vi "4-2-1 Chemical Process Monitoring.vi"() -> ()   [LabVIEW 2020]
uses:
  state.ctl
  <vilib>/addons/WebSockets-API-master/WebSockets/WebSocket Client/WebSocket Client.lvclass
  C:/Program Files (x86)/National Instruments/LabVIEW 2020/vi.lib/addons/WebSockets-API-master/WebSockets/WebSocket/WebSocket.lvclass
  <vilib>/addons/WebSockets-API-master/WebSockets/WebSocket/WebSocket.lvclass
panel:
  out "Read Data":string
  in  "Stop":bool
  out "connection error?":bool
  in  "sensor_data":T1={"temp_reactor"=60.0, "temp_coolant"=25.0, "press_reactor"=1.2, "stir_speed"=220.0, "coolant_flow"=TRUE, "exhaust_valve"=FALSE, "timestamp"="21:38:10"}
  out "connect?":bool
  in  "WebSockets URL":string="ws://localhost:8000/ws/labview"
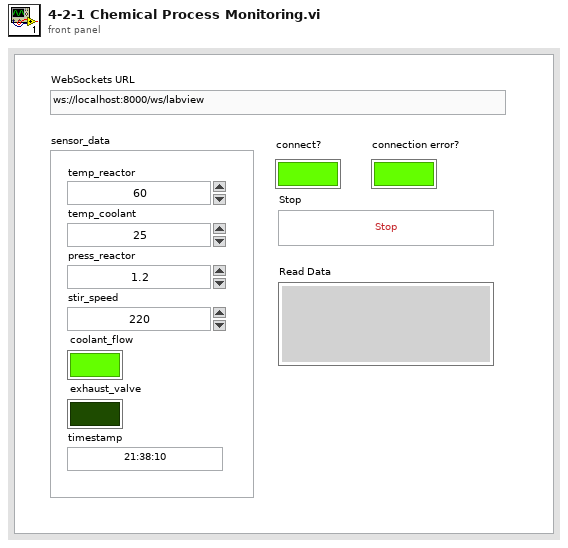
[diagram p1: front panel]
types:
  T1 = cluster{"temp_reactor":dbl, "temp_coolant":dbl, "press_reactor":dbl, "stir_speed":dbl, "coolant_flow":bool, "exhaust_valve":bool, "timestamp":string}
  T2 = typedef "state.ctl" = enum16{"CONNECT", "WRITE_DATA", "READ_DATA", "DISCONNECT"}
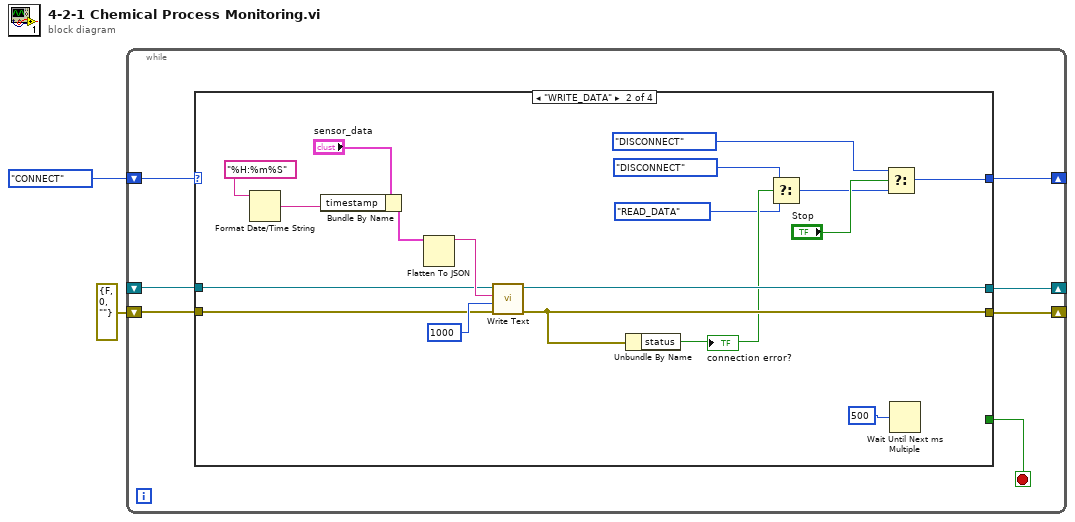
[diagram p0: block diagram]
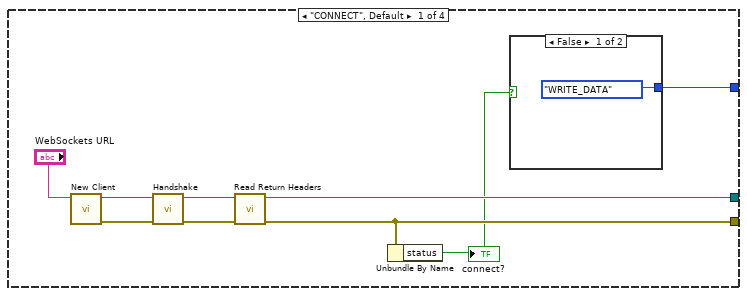
[diagram p2: hidden frame]
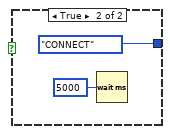
[diagram p3: hidden frame]
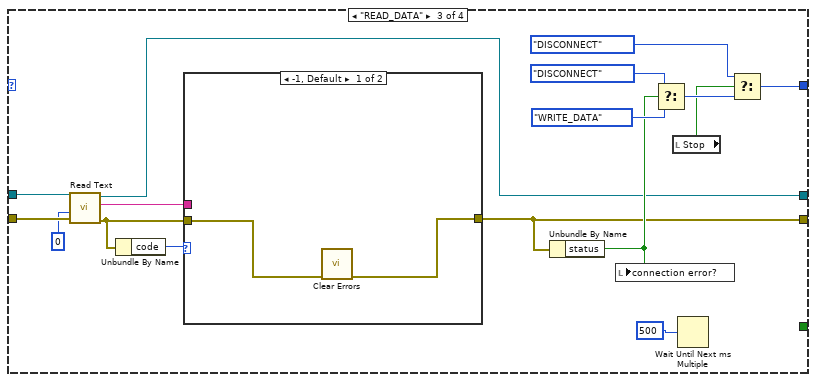
[diagram p4: hidden frame]
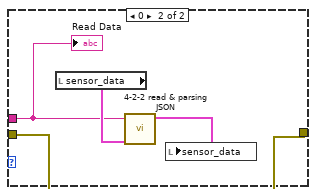
[diagram p5: hidden frame]
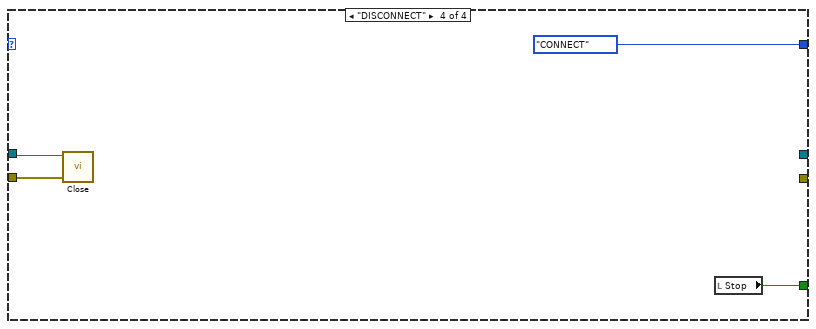
[diagram p6: hidden frame]
diagram:
  n1 = while {
    shift-right: [w6] -> _
    shift-left: state."CONNECT" -> [w9]
    shift-right: [w8] -> _
    shift-left: _ -> [w5]
    shift-right: [w7] -> _
    shift-left: errorcluster {"status"=FALSE, "code"=0, "source"=""} ("error out") -> [w4]
    stop <- w3 stop-if-true
    n2 = case shown="\"WRITE_DATA\"" w9 {
      tunnel: [w13 w35 w41 _] -> w8
      tunnel: [w12 w34 w42 _] -> w7
      tunnel: [w10 w26 w51 state."CONNECT"] -> w6
      tunnel: w5 -> [_ w37 w48 w65]
      tunnel: w4 -> [_ w36 w47 w64]
      tunnel: [_ _ _ w63] -> w3
      frame "CONNECT", Default {
        n3 = call <vilib>:"New Client.vi"("WebSocket URL"="WebSockets URL") -> ("error out"=w14:errorcluster, "WebSocket Client out"=w16:refnum<class "WebSocket Client.lvclass">)  [unwired: 9 in]
        n4 = call-dynamic "Handshake.vi"("error in (no error)"=w14, "WebSocket Client in"=w16) -> ("error out"=w17:errorcluster, "WebSocket Client out"=w18:refnum<class "WebSocket Client.lvclass">)  [unwired: 8 in]
        n5 = call <vilib>:"Read Return Headers.vi"("error in (no error)"=w17, "WebSocket in"=w18) -> ("error out"=w12:errorcluster, "WebSocket out"=w13:refnum<class "WebSocket Client.lvclass">)  [unwired: 7 in, 1 out]
        n6 = Unbundle By Name(w12) -> ("status"=w11:bool)
        "connect?" <- w11
        n7 = case shown="False" w11 {
          tunnel: [state."WRITE_DATA" state."CONNECT"] -> w10
          frame False {
          }
          frame True {
            n8 = Wait (ms)(milliseconds to wait=u32 5000) -> ()  [unwired: 1 out]
          }
        }
      }
      frame "WRITE_DATA" {
        n9 = Format Date/Time String(time format string (%c)="%H:%m%S") -> (date/time string=w23:string)  [unwired: 2 in]
        n10 = Bundle By Name(cluster="sensor_data", "timestamp"=w23) -> (w22:T1)
        n11 = Flatten To JSON(anything=w22) -> (JSON string=w39:string)  [unwired: 2 in, 1 out]
        n12 = call-dynamic "Write Text.vi"("error in (no error)"=w36, "timeout ms (5000)"=1000, "String Data"=w39, "WebSocket in"=w37) -> ("error out"=w34:errorcluster, "WebSocket out"=w35:refnum<class "WebSocket.lvclass">)  [unwired: 6 in]
        n13 = Unbundle By Name(w34) -> ("status"=w32:bool)
        "connection error?" <- w32
        n14 = Select(t=state."DISCONNECT", s=w32, f=state."READ_DATA") -> (s? t:f=w28:T2)
        n15 = Select(t=state."DISCONNECT", s="Stop", f=w28) -> (s? t:f=w26:T2)
        n16 = Wait Until Next ms Multiple(millisecond multiple=u32 500) -> ()  [unwired: 1 out]
      }
      frame "READ_DATA" {
        n17 = call-dynamic "Read Text.vi"("error in (no error)"=w47, "timeout ms (5000)"=0, "WebSocket in"=w48) -> ("error out"=w43:errorcluster, "Data"=w44:string, "WebSocket out"=w41:refnum<class "WebSocket.lvclass">)  [unwired: 6 in]
        n18 = Unbundle By Name(w43) -> ("code"=w45:i32)
        n19 = case shown="-1, Default" w45 {
          tunnel: w44 -> [_ w58]
          tunnel: w43 -> [w57 w59]
          tunnel: [w56 w59] -> w42
          frame -1, Default {
            n20 = call <vilib>:"Clear Errors.vi"("error in (no error)"=w57) -> ("error out"=w56:errorcluster)  [unwired: 5 in, 1 out]
          }
          frame 0 {
            n21 = local read "sensor_data"() -> (w61:T1)
            n22 = call "4-2-2 read & parsing JSON.vi"("sensor_data"=w61, "read JSON data"=w58) -> ("sensor_data out"=w60:T1)  [unwired: 9 in]
            n23 = local write "sensor_data"(w60) -> ()
            "Read Data" <- w58
          }
        }
        n24 = Unbundle By Name(w42) -> ("status"=w49:bool)
        n25 = local write "connection error?"(w49) -> ()
        n26 = Select(t=state."DISCONNECT", s=w49, f=state."WRITE_DATA") -> (s? t:f=w53:T2)
        n27 = local read "Stop"() -> (w50:bool)
        n28 = Wait Until Next ms Multiple(millisecond multiple=u32 500) -> ()  [unwired: 1 out]
        n29 = Select(t=state."DISCONNECT", s=w50, f=w53) -> (s? t:f=w51:T2)
      }
      frame "DISCONNECT" {
        n30 = call-dynamic "Close.vi"("error in (no error)"=w64, "WebSocket in"=w65) -> ()  [unwired: 9 in, 1 out]
        n31 = local read "Stop"() -> (w63:bool)
      }
    }
  }
